vi "SetHold.vi"(6 "Legacy (f)?":bool, 8 "error in (no error)":errorcluster, 10 "Hold":bool) -> (0 "error out":errorcluster)   [LabVIEW 2011]
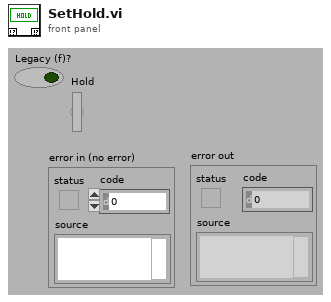
[diagram p1: front panel]
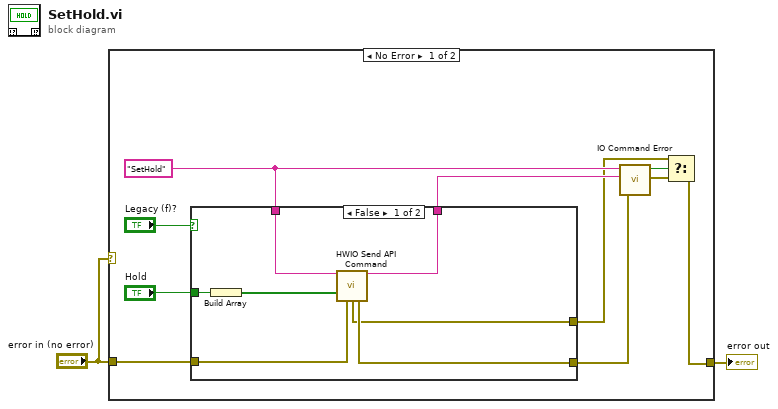
[diagram p0: block diagram]
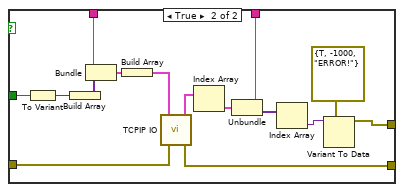
[diagram p2: hidden frame]
diagram:
  n1 = case shown="No Error" "error in (no error)" {
    tunnel: "error in (no error)" -> [w11 w35]
    tunnel: [w4 w35] -> w2
    frame No Error {
      w9 = "SetHold"
      n2 = case shown="False" "Legacy (f)?" {
        tunnel: "Hold" -> [w15 w34]
        tunnel: w11 -> [w19 w31]
        tunnel: [w18 w29] -> w10
        tunnel: w9 -> [w16 w28]
        tunnel: [w17 w25] -> w8
        tunnel: [w13 w21] -> w7
        frame False {
          n3 = Build Array(w15) -> (w14:bool[])
          n4 = call "HWIO Send API Command.vi"("Action"=w16, "Boolean"=w14, "error in (no error)"=w19) -> ("Action out"=w17:string, "HWError"=w13:errorcluster, "error out"=w18:errorcluster)  [unwired: 5 in, 5 out]
        }
        frame True {
          n5 = To Variant(anything=w34) -> (Variant=w33:variant)
          n6 = Build Array(w33) -> (w32:variant[])
          n7 = Bundle(w28, w32) -> (w30:cluster{string, variant[]})  [unwired: 1 out]
          n8 = Build Array(w30) -> (w27:cluster{string, variant[]}[])
          n9 = call "TCPIP IO.vi"("error in (no error)"=w31, "Commands"=w27) -> ("error out"=w29:errorcluster, "Responses"=w24:cluster{string, variant[]}[])  [unwired: 1 in, 3 out]
          n10 = Index Array(array=w24) -> (element=w26:cluster{string, variant[]})  [unwired: 1 in]
          n11 = Unbundle(w26) -> (w25:string, w20:variant[])
          n12 = Index Array(array=w20) -> (element=w23:variant)  [unwired: 1 in]
          n13 = Variant To Data(type=errorcluster {"status"=TRUE, "code"=-1000, "source"="ERROR!"} ("error out"), Variant=w23) -> (data=w21:errorcluster)  [unwired: 1 in, 1 out]
        }
      }
      n14 = call "IO Command Error.vi"("error in (no error)"=w10, "Command Returned (\"\")"=w8, "Command Sent (\"\")"=w9) -> ("error out"=w5:errorcluster, "HW ERR?"=w6:bool)  [unwired: 3 out]
      n15 = Select(t=w7, s=w6, f=w5) -> (s? t:f=w4:errorcluster)
    }
    frame Error {
    }
  }
  "error out" <- w2
